vi "SysIdRoutine_Close.vi"(7 "dir":string, 11 "in SysIdRoutine":T3={"m_config"={"m_timeout_Sec"=10.0, "m_stepVoltage_Volt"=7.0, "m_rampRate_V/S"=1.0}, "m_mechanism"={"m_drive_volts"=0.0, "m_log"=[], "m_name"=""}, "m_outputVolts"=0.0, "m_recordState"=enum."kNone", "timer"={"StartTime"=0.0, "Accumulated TIme"=0.0, "Running"=FALSE, "semaphore"=refnum}} {"timer"."Accumulated TIme" format="%13.5p"; "timer"."StartTime" format="%13.5p"}) -> (4 "Full Filename":string)   [LabVIEW 2023]
uses:
  <vilib>/Rock Robotics/WPI/ThirdParty/JAS_Junk/TrajLib/TypeDef/TIMER.ctl
  impl_ControlRecordType_ENUM.ctl
  <vilib>/Rock Robotics/WPI/ThirdParty/JAS_Junk/TrajLib/Trajectory_Library.lvlib
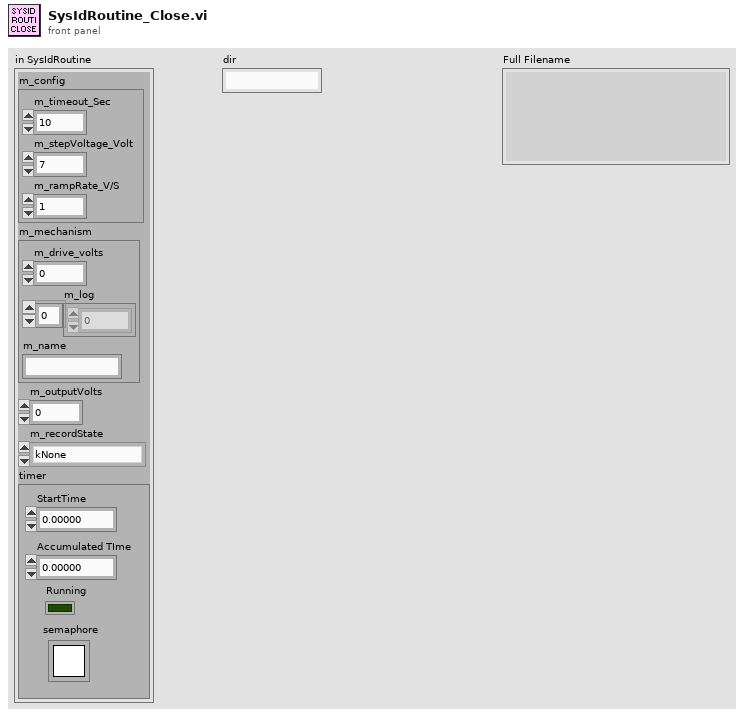
[diagram p1: front panel]
types:
  T1 = typedef "Trajectory_Library.lvlib/TIMER.ctl" = cluster{"StartTime":dbl, "Accumulated TIme":dbl, "Running":bool, "semaphore":T2}
  T2 = typedef "Semaphore RefNum" = refnum<k1>
  T3 = cluster{"m_config":cluster{"m_timeout_Sec":dbl, "m_stepVoltage_Volt":dbl, "m_rampRate_V/S":dbl}, "m_mechanism":cluster{"m_drive_volts":dbl, "m_log":u8[], "m_name":string}, "m_outputVolts":dbl, "m_recordState":enum16{"kQuasistaticForward", "kQuasistaticReverse", "kDynamicForward", "kDynamicReverse", "kNone"}, "timer":T1}
  T4 = enum16{"big-endian, network order", "native, host order", "little-endian"}
  T5 = typedef "impl_ControlRecordType_ENUM.ctl" = enum16{"kControlStart", "kControlFinish", "kControlSetMetadata"}
  T6 = cluster{"entry ID being started/completed/updated":i32, "entry name UTF-8 string data (arbitrary length)":string, "entry type UTF-8 string data (arbitrary length)":string, "entry metadata UTF-8 string data (arbitrary length)":string}
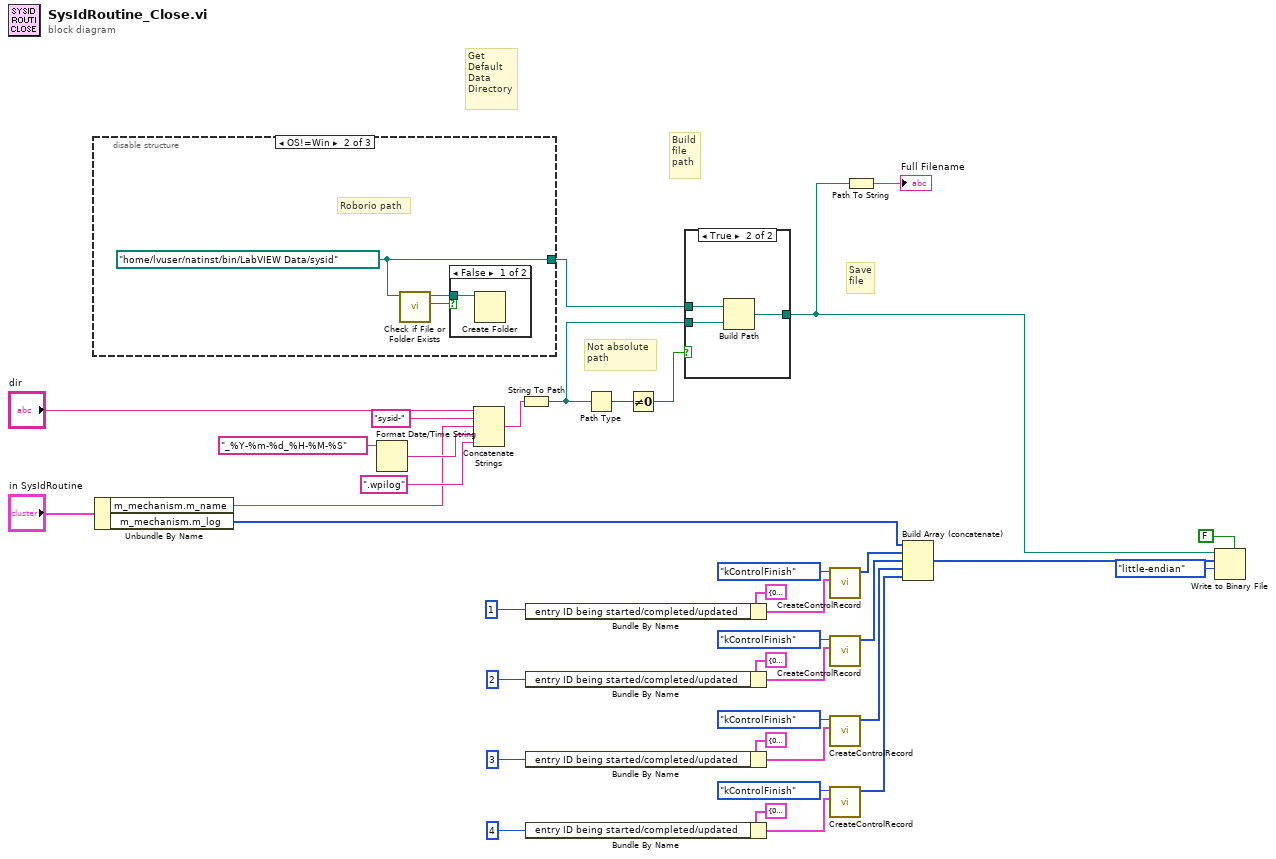
[diagram p0: block diagram]
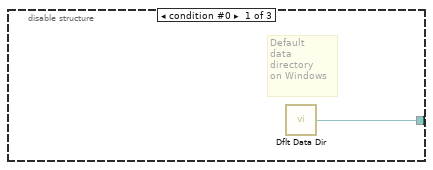
[diagram p3: hidden frame]
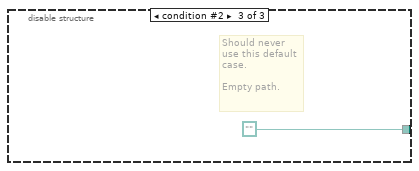
[diagram p5: hidden frame]
diagram:
  # "Not absolute\npath"
  # "Get\nDefault\nData\nDirectory"
  # "Save\nfile"
  # "Build\nfile\npath"
  n1 = disable-structure shown="OS!=Win" {
    disable-tunnel: [w39 w41 path ""] -> w13
    frame condition #0 {
      # "Default\ndata\ndirectory\non Windows"
      n2 = call <vilib>:"Dflt Data Dir.vi"() -> ("App:Default Data Directory"=w39:path)
    }
    frame condition #1 (active) {
      w41 = path "/home/lvuser/natinst/bin/LabVIEW Data/sysid"
      # "Roborio path"
      n3 = call <vilib>:"Check if File or Folder Exists.vi"("path"=w41) -> ("file or folder exists?"=w40:bool, "dup path"=w42:path)  [unwired: 8 in, 1 out]
      n4 = case shown="False" w40 {
        tunnel: w42 -> [w43 _]
        frame False {
          n5 = Create Folder(path (use dialog)=w43) -> ()  [unwired: 2 in, 3 out]
        }
        frame True {
        }
      }
    }
    frame condition #2 {
      # "Should never\nuse this default\ncase.\n\nEmpty path."
    }
  }
  n6 = Unbundle By Name("in SysIdRoutine") -> ("m_mechanism.m_name"=w2:string, "m_mechanism.m_log"=w14:u8[])
  n7 = Format Date/Time String(time format string (%c)="_%Y-%m-%d_%H-%M-%S") -> (date/time string=w6:string)  [unwired: 2 in]
  n8 = Concatenate Strings("dir", "sysid-" ("string"), w2, w6, ".wpilog" ("string")) -> (w4:string)
  n9 = String To Path(string=w4) -> (path=w12:path)
  n10 = Bundle By Name(cluster=T6 {"entry ID being started/completed/updated"=0, "entry name UTF-8 string data (arbitrary length)"="", "entry type UTF-8 string data (arbitrary length)"="", "entry metadata UTF-8 string data (arbitrary length)"=""} ("Control Record Payload Data"), "entry ID being started/completed/updated"=1) -> (w29:T6)
  n11 = Bundle By Name(cluster=T6 {"entry ID being started/completed/updated"=0, "entry name UTF-8 string data (arbitrary length)"="", "entry type UTF-8 string data (arbitrary length)"="", "entry metadata UTF-8 string data (arbitrary length)"=""} ("Control Record Payload Data"), "entry ID being started/completed/updated"=2) -> (w30:T6)
  n12 = Bundle By Name(cluster=T6 {"entry ID being started/completed/updated"=0, "entry name UTF-8 string data (arbitrary length)"="", "entry type UTF-8 string data (arbitrary length)"="", "entry metadata UTF-8 string data (arbitrary length)"=""} ("Control Record Payload Data"), "entry ID being started/completed/updated"=3) -> (w32:T6)
  n13 = Bundle By Name(cluster=T6 {"entry ID being started/completed/updated"=0, "entry name UTF-8 string data (arbitrary length)"="", "entry type UTF-8 string data (arbitrary length)"="", "entry metadata UTF-8 string data (arbitrary length)"=""} ("Control Record Payload Data"), "entry ID being started/completed/updated"=4) -> (w31:T6)
  n14 = Path Type(1:w12) -> (0:w11:i16)
  n15 = Not Equal To 0?(x=w11) -> (x != 0?=w10:bool)
  n16 = case shown="True" w10 {
    tunnel: [w45 w48] -> w8
    tunnel: w13 -> [_ w47]
    tunnel: w12 -> [w45 w46]
    frame False {
    }
    frame True {
      n17 = Build Path(base path=w47, name or relative path=w46) -> (appended path=w48:path)
    }
  }
  n18 = call "CreateControlRecord.vi"("Control Record Payload Data"=w29, "ControlRecordType"=impl_ControlRecordType_ENUM."kControlFinish") -> ("control record"=w33:u8[])  [unwired: 9 in]
  n19 = call "CreateControlRecord.vi"("Control Record Payload Data"=w30, "ControlRecordType"=impl_ControlRecordType_ENUM."kControlFinish") -> ("control record"=w34:u8[])  [unwired: 9 in]
  n20 = call "CreateControlRecord.vi"("Control Record Payload Data"=w32, "ControlRecordType"=impl_ControlRecordType_ENUM."kControlFinish") -> ("control record"=w35:u8[])  [unwired: 9 in]
  n21 = call "CreateControlRecord.vi"("Control Record Payload Data"=w31, "ControlRecordType"=impl_ControlRecordType_ENUM."kControlFinish") -> ("control record"=w36:u8[])  [unwired: 9 in]
  n22 = Path To String(path=w8) -> (string=→"Full Filename":string)
  n23 = Build Array (concatenate)(w14, w33, w34, w35, w36) -> (w37:u8[])
  n24 = Write to Binary File(file (use dialog)=w8, data=w37, 5:FALSE ("prepend array or string size? (T)"), 9:T4."little-endian" ("byte order (0:big-endian, network order)")) -> ()  [unwired: 2 in, 3 out]
